vi "mod_Rician Fading (Jakes).vi"(0 "profile length (samples)":i32=1000, 1 "rician parameter K (dB)":dbl=1.0 format="%.2f", 5 "sampling frequency (Hz)":dbl=1.0 format="%.2f", 7 "doppler spread (Hz)":dbl=0.01 format="%.2p", 9 "seed in (0xFFFFFFFF)":i32=-1 format="%.0x", 11 "error in (no error)":errorcluster, 12 "fading variance":dbl=1.0 format="%.2f", 13 "reset? (T)":bool=TRUE) -> (4 "rician fading profile":cdb[](array[numeric]) format="%.2f", 10 "next seed":i32=-1 format="%.0x", 15 "error out":errorcluster)   [LabVIEW 2020, in "niDMT.lvlib"]
doc: "The Rayleigh fading channel is generated based on Clarke and Gans Model using the Doppler filter with U-shaped power spectral density. \n \n\n Inputs:\n 1) Doppler spread (Hz) \n - range : double precision (default:20)\n - an example : a running vehicle with 65mph (104km/h), the carrier frequency of 900MHz\n The speed of the vehicle = 65*1.6*1000/3600 = 28.89m/s\n Doppler frequency = (900MHz)*(28.89m/s)/(300*10^6m/s) = 86.67 Hz\n 2) Fading variance : the variance of the fading channel output\n - range : double precision (default:2)\n 3) Input waveform : Input signal samples\n - some default values were set.\n (dt:0.00025, the number of samples:4000)\n 4) seed in (0xFFFFFFFF)\n 5) Error in\n\n Outputs:\n 1) Rayleigh fading profile : the complex fading channel output\n 2) Error out"
uses:
  <vilib>/addons/Modulation/niDMT.lvlib
  <vilib>/addons/Modulation/niAMT.lvlib
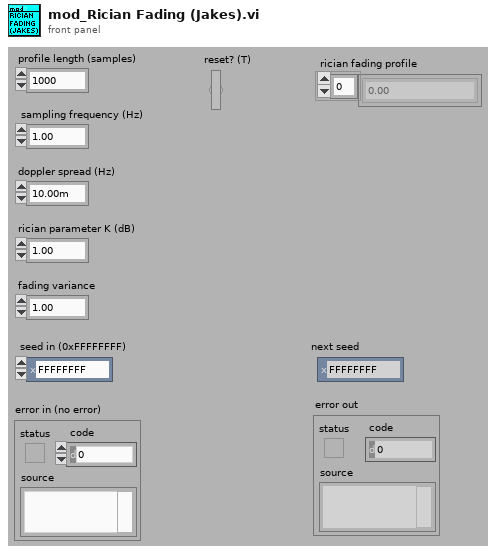
[diagram p1: front panel]
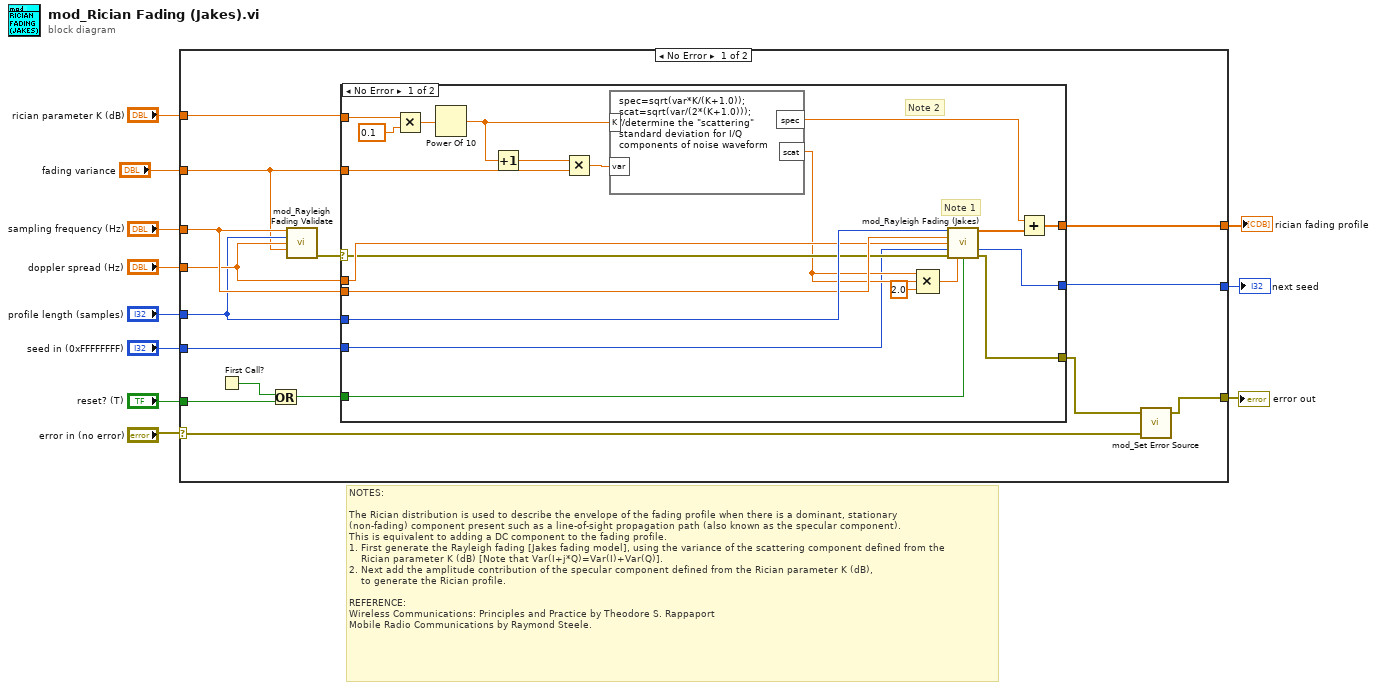
[diagram p0: block diagram]
diagram:
  # "NOTES:\n\nThe Rician distribution is used to describe the envelope of the fading profile when there is a dominant, stationary\n(non-fading) component present such as a line-of-sight propagation path (also known as the specular component).\nThis is equivalent to adding a DC component to the fading profile.\n1. First generate the Rayleigh fading [Jakes fading model], using the variance of the scattering component defined from the\n    Rician parameter K (dB) [Note that Var(I+j*Q)=Var(I)+Var(Q)].\n2. Next add the amplitude contribution of the specular component defined from the Rician parameter K (dB),\n    to generate the Rician profile.\n\nREFERENCE:\nWireless Communications: Principles and Practice by Theodore S. Rappaport\nMobile Radio Communications by Raymond Steele."
  n1 = case shown="No Error" "error in (no error)" {
    selector: "error in (no error)" -> [w25 w49]
    tunnel: [w26 w49] -> w11
    tunnel: [w21 _] -> w9
    tunnel: "rician parameter K (dB)" -> [w13 _]
    tunnel: "sampling frequency (Hz)" -> [w20 _]
    tunnel: "doppler spread (Hz)" -> [w19 _]
    tunnel: "profile length (samples)" -> [w18 _]
    tunnel: "seed in (0xFFFFFFFF)" -> [w17 _]
    tunnel: "reset? (T)" -> [w15 _]
    tunnel: "fading variance" -> [w14 _]
    tunnel: [w12 _] -> w1
    frame No Error {
      n2 = First Call?() -> (First Call?: T/F=w16:bool)
      n3 = Or(x=w16, y=w15) -> (x .or. y?=w22:bool)
      n4 = call <vilib>:"mod_Rayleigh Fading Validate.vi"("sampling frequency"=w20, "profile length (samples)"=w18, "doppler spread (Hz)"=w19, "fading variance"=w14) -> ("error out"=w23:errorcluster)  [unwired: 1 in, 10 out]
      n5 = case shown="No Error" w23 {
        selector: w23 -> [w41 w48]
        tunnel: w19 -> [w42 _]
        tunnel: w18 -> [w44 _]
        tunnel: [w33 w48] -> w24
        tunnel: w20 -> [w43 _]
        tunnel: w13 -> [w45 _]
        tunnel: w22 -> [w37 _]
        tunnel: [w34 _] -> w21
        tunnel: w17 -> [w32 _]
        tunnel: w14 -> [w28 _]
        tunnel: [w31 _] -> w12
        frame No Error {
          # "Note 2"
          # "Note 1"
          n6 = Multiply(x=w45, y=0.1) -> (x*y=w47:dbl)
          n7 = Power Of 10(x=w47) -> (10^x=w30:dbl)
          n8 = Increment(x=w30) -> (x+1=w29:dbl)
          n9 = Multiply(x=w29, y=w28) -> (x*y=w27:dbl)
          n10 = formula code="spec=sqrt(var*K/(K+1.0));\nscat=sqrt(var/(2*(K+1.0)));\n//determine the \"scattering\" standard deviation for I/Q components of noise waveform"("K"=w30, "var"=w27) -> ("scat"=w40:dbl, "spec"=w35:dbl)
          n11 = Compound Arithmetic op=MULTIPLY(w40, w40, 2.0 ("value")) -> (w39:dbl)
          n12 = call <vilib>:"mod_Rayleigh Fading (Jakes).vi"("profile length (samples)"=w44, "sampling frequency (Hz)"=w43, "doppler spread (Hz)"=w42, "seed in (0xFFFFFFFF)"=w32, "error in (no error)"=w41, "fading variance"=w39, "reset? (T)"=w37) -> ("rayleigh fading profile"=w36:cdb[], "next seed"=w31:i32, "error out"=w33:errorcluster)  [unwired: 6 out]
          n13 = Add(x=w35, y=w36) -> (x+y=w34:cdb[])
        }
        frame Error {
        }
      }
      n14 = call <vilib>:"mod_Set Error Source.vi"("initial error in (no error)"=w25, "final error in (no error)"=w24) -> ("error out"=w26:errorcluster)  [unwired: 1 in, 2 out]
    }
    frame Error {
    }
  }
  "error out" <- w11
  "rician fading profile" <- w9
  "next seed" <- w1
